vi "pp2_DAQwriteAudioStimulus.vi"(0 "State Info In":T4={"Curr  tr"=0, "Curr (ms)"=0, "Cum (ms)"=0, "Run loop diff"=0, "Tone countdown (ms)"=0, "Countdown (ms)"=0, "Curr State"=enum."0 NULL", "Prev State"=enum."1 Habituation", "Null"=FALSE, "Sw"=FALSE, "Tone\nGate"=FALSE, "Stim"=FALSE, "Current DAQ DO Int"=0, "Current Loaded Trial"={"Trial Type Number"=1, "Trial Type"=enum."GO", "Trial Weight"=100, "Shock (mA)"=0.3, "Duration (ms)"=0.25, "Sound Type"=enum."04 FM Sweep", "Stim P1"=4000.0, "Stim P2"=0.0, "Stim P3"=0.0, "Stim P4"=2000.0}, "Next Trial (for display purposes)"={"Trial Type Number"=1, "Trial Type"=enum."GO", "Trial Weight"=100, "Shock (mA)"=0.3, "Duration (ms)"=0.25, "Sound Type"=enum."04 FM Sweep", "Stim P1"=4000.0, "Stim P2"=0.0, "Stim P3"=0.0, "Stim P4"=2000.0}, "Total trials memo"=0, "State start cum memo (ms)"=0, "Last dur jump time memo (ms)"=0, "Last dur shock time memo (ms)"=0, "Tone repeat memo (ms)"=0, "Webcam on"=FALSE, "Webcam recording"=FALSE} {"Current DAQ DO Int" format="%b"; "Next Trial (for display purposes)"."Shock (mA)" min=-1.0 max=5.0; "Next Trial (for display purposes)"."Trial Weight" step=1; "Next Trial (for display purposes)"."Duration (ms)" min=0.0 max=1.0; "Next Trial (for display purposes)"."Trial Type Number" min=1 step=1; "Current Loaded Trial"."Shock (mA)" min=-1.0 max=5.0; "Current Loaded Trial"."Trial Weight" step=1; "Current Loaded Trial"."Duration (ms)" min=0.0 max=1.0; "Current Loaded Trial"."Trial Type Number" min=1 step=1}, 5 "Daq config In":T1={"Sound AO"="Dev2/ao0", "Shock intesity AO"="Dev1/ao1", "Code_LED DO"="Dev1/port1:2", "Switch DI"="Dev1/port0/line0:1", "Webcam"="cam0", "Sound AO task"="", "Sound card task"=0, "Shock intensity AO task"="", "Code_LED DO task"="", "Switch DI task"="", "AO <=> Sound card"=FALSE, "Sound card"=0, "sample rate"=8000.0, "Variable shock"=FALSE, "Webcam on"=FALSE, "Tone gate PFI"="/Dev1/PFI1", "Waveform memo"={"t0"=timestamp(0 s since 1904-01-01), "dt"=1.0, "Y"=[]}} {"sample rate" min=8000.0; "Sound card task" format="%.0x"}, 11 "error in (no error)":errorcluster) -> (6 "Daq config Out":T1={"Sound AO"="Dev2/ao0", "Shock intesity AO"="Dev1/ao1", "Code_LED DO"="Dev1/port1:2", "Switch DI"="Dev1/port0/line0:1", "Webcam"="cam0", "Sound AO task"="", "Sound card task"=0, "Shock intensity AO task"="", "Code_LED DO task"="", "Switch DI task"="", "AO <=> Sound card"=FALSE, "Sound card"=0, "sample rate"=8000.0, "Variable shock"=FALSE, "Webcam on"=FALSE, "Tone gate PFI"="/Dev1/PFI1", "Waveform memo"={"t0"=timestamp(0 s since 1904-01-01), "dt"=1.0, "Y"=[]}} {"sample rate" min=8000.0; "Sound card task" format="%.0x"}, 15 "error out":errorcluster)   [LabVIEW 2013]
uses:
  pp2_CTL_StateInfo.ctl
  pp2_CTL_State.ctl
  pp2_Trial.ctl
  pp2_CTL_TrialType.ctl
  labolabo2/waveforms/WFTypes.ctl
  pp2_CTL_DaqConfig.ctl
  <vilib>/userdefined/High Color/IMAQdx.ctl
  <vilib>/sound2/lvsound2.llb/Sound Output Task ID.ctl
  labolabo2/waveforms/WFParameters.ctl
  labolabo2/waveforms/WFRepetitions.ctl
  <vilib>/Analysis/NI_AALBase.lvlib
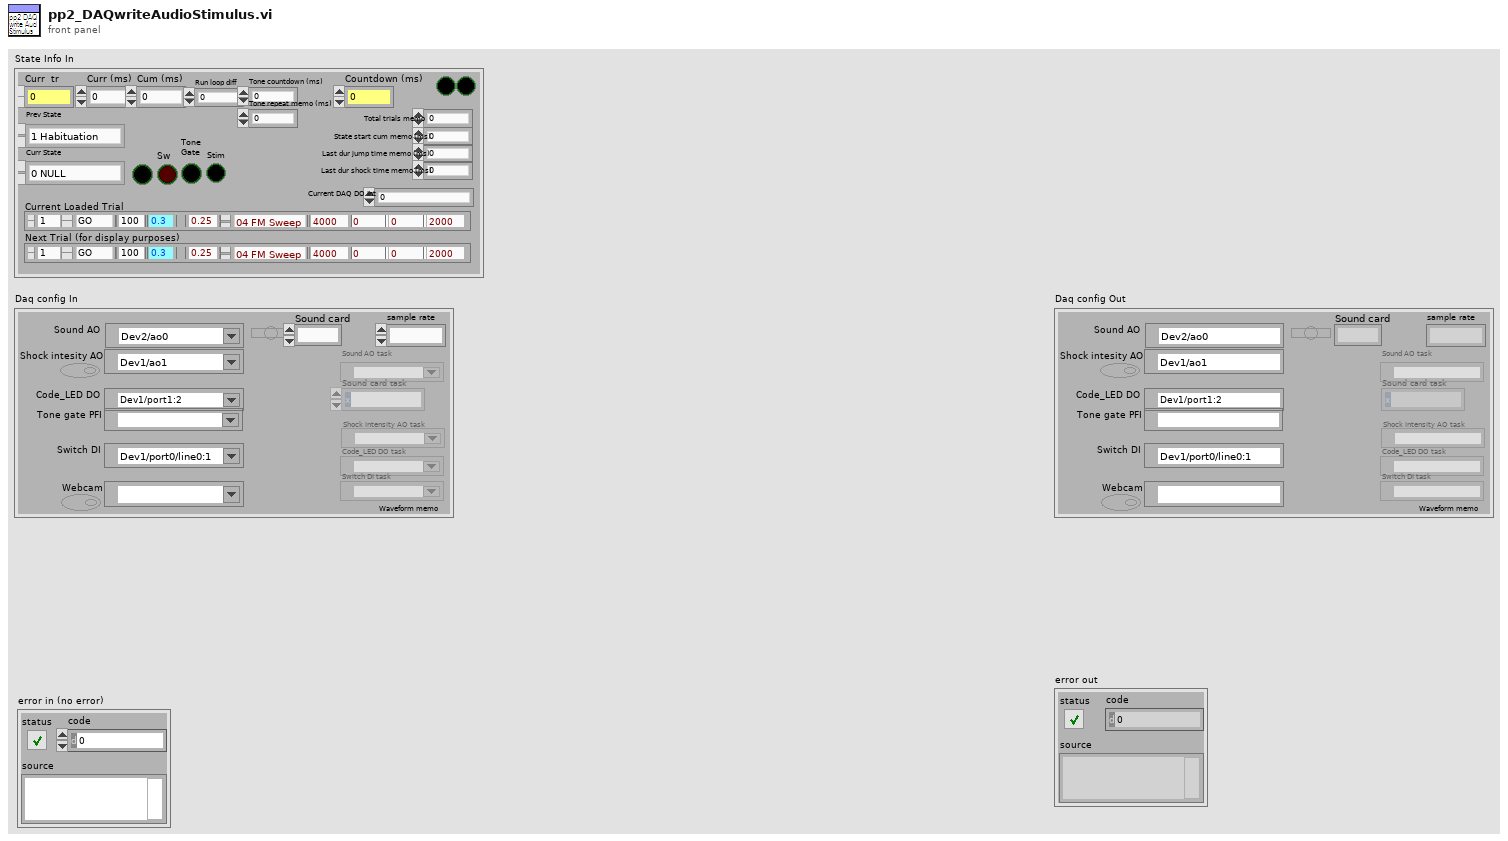
[diagram p1: front panel]
types:
  T1 = typedef "pp2_CTL_DaqConfig.ctl" = cluster{"Sound AO":tag, "Shock intesity AO":tag, "Code_LED DO":tag, "Switch DI":tag, "Webcam":T2, "Sound AO task":refnum<k21>, "Sound card task":T3, "Shock intensity AO task":refnum<k21>, "Code_LED DO task":refnum<k21>, "Switch DI task":refnum<k21>, "AO <=> Sound card":bool, "Sound card":u32, "sample rate":dbl, "Variable shock":bool, "Webcam on":bool, "Tone gate PFI":tag, "Waveform memo":waveform(dbl)}
  T2 = typedef "IMAQdx.ctl" = refnum<k21>
  T3 = typedef "Sound Output Task ID.ctl" = u32
  T4 = typedef "pp2_CTL_StateInfo.ctl" = cluster{"Curr  tr":u16, "Curr (ms)":u32, "Cum (ms)":i64, "Run loop diff":i64, "Tone countdown (ms)":i64, "Countdown (ms)":i64, "Curr State":T5, "Prev State":T5, "Null":bool, "Sw":bool, "Tone\nGate":bool, "Stim":bool, "Current DAQ DO Int":u16, "Current Loaded Trial":T6, "Next Trial (for display purposes)":T6, "Total trials memo":i64, "State start cum memo (ms)":i64, "Last dur jump time memo (ms)":i64, "Last dur shock time memo (ms)":i64, "Tone repeat memo (ms)":i64, "Webcam on":bool, "Webcam recording":bool}
  T5 = typedef "pp2_CTL_State.ctl" = enum8{"0 NULL", "1 Habituation", "2 (Load Trial)", "3 Stay Period", "4 Load Audio/Click Delay", "5 GO Trial", "6 GO Jumped", "7 GO Timeout", "8 NOGO Trial", "9 NOGO Jumped", "10 NOGO Timeout", "11 TEST Trial", "12 TEST Jumped", "13 TEST Timeout", "14 Intertrial Interval", "15 Done"}
  T6 = typedef "pp2_Trial.ctl" = cluster{"Trial Type Number":u8, "Trial Type":T7, "Trial Weight":u32, "Shock (mA)":dbl, "Duration (ms)":dbl, "Sound Type":T8, "Stim P1":dbl, "Stim P2":dbl, "Stim P3":dbl, "Stim P4":dbl}
  T7 = typedef "pp2_CTL_TrialType.ctl" = enum16{"OFF", "GO", "NOGO", "TEST"}
  T8 = typedef "WFTypes.ctl" = enum16{"00 NULL", "01 DC", "02 Noise", "03 Pure Tone", "04 FM Sweep"}
  T9 = typedef "WFRepetitions.ctl" = cluster{"Del (s)":dbl, "Int (s)":dbl, "N":i32}
  T10 = typedef "WFParameters.ctl" = cluster{"Fs (Hz)":dbl, "Amp (V)":dbl, "Ramp (s)":dbl, "Dur (s)":dbl}
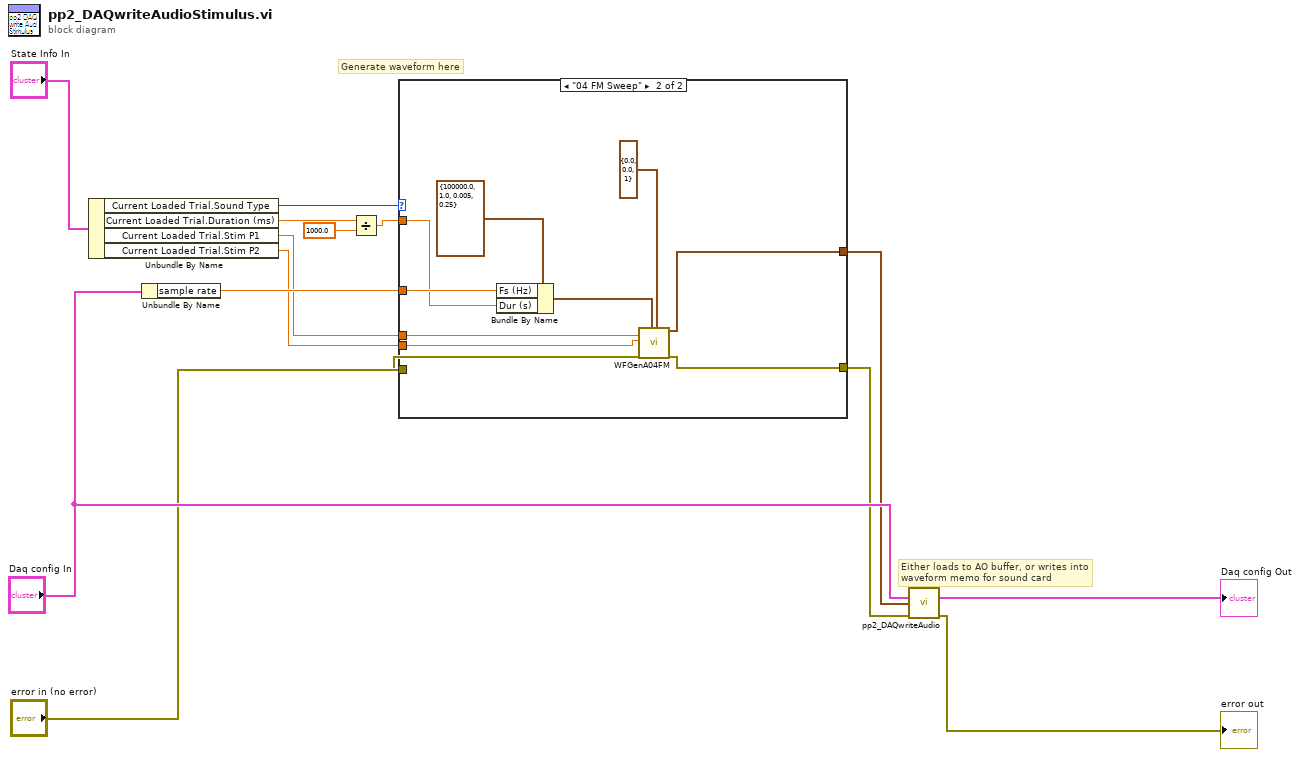
[diagram p0: block diagram]
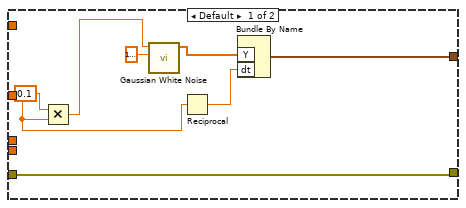
[diagram p2: hidden frame]
diagram:
  # "Either loads to AO buffer, or writes into\nwaveform memo for sound card"
  # "Generate waveform here"
  n1 = Unbundle By Name("State Info In") -> ("Current Loaded Trial.Sound Type"=w13:T8, "Current Loaded Trial.Duration (ms)"=w3:dbl, "Current Loaded Trial.Stim P1"=w5:dbl, "Current Loaded Trial.Stim P2"=w4:dbl)
  n2 = Unbundle By Name("Daq config In") -> ("sample rate"=w12:dbl)
  n3 = Divide(x=w3, y=1000.0) -> (x/y=w2:dbl)
  n4 = case shown="\"04 FM Sweep\"" w13 {
    tunnel: w12 -> [w17 w31]
    tunnel: [w16 w24] -> w7
    tunnel: "error in (no error)" -> [w15 w25]
    tunnel: [w15 w23] -> w9
    tunnel: w2 -> [_ w28]
    tunnel: w5 -> [_ w27]
    tunnel: w4 -> [_ w26]
    frame Default {
      n5 = Multiply(x=0.1, y=w17) -> (x*y=w20:dbl)
      n6 = call <vilib>:"Gaussian White Noise.vi"("standard deviation"=1.0000000000000002, "samples"=w20) -> ("Gaussian noise pattern"=w19:dbl[])  [unwired: 8 in, 1 out]
      n7 = Reciprocal(x=w17) -> (1/x=w18:dbl)
      n8 = Bundle By Name("Y"=w19, "dt"=w18) -> (w16:waveform(dbl))  [unwired: 1 in]
    }
    frame "04 FM Sweep" {
      n9 = Bundle By Name(cluster=T10 {"Fs (Hz)"=100000.0, "Amp (V)"=1.0, "Ramp (s)"=0.005, "Dur (s)"=0.25} ("WFParameters"), "Fs (Hz)"=w31, "Dur (s)"=w28) -> (w29:T10)
      n10 = call "WFGenA04FM.vi"("Param 0: Start Hz"=w27, "Param 1: End Hz"=w26, "error in (no error)"=w25, "WFParameters"=w29, "WFRepetitions"=T9 {"Del (s)"=0.0, "Int (s)"=0.0, "N"=1}) -> ("Waveform Out"=w24:waveform(dbl), "error out"=w23:errorcluster)  [unwired: 13 in]
    }
  }
  n11 = call "pp2_DAQwriteAudio.vi"("Daq config In"="Daq config In", "Waveform"=w7, "error in (no error)"=w9) -> ("Daq config Out"=→"Daq config Out":T1, "error out"=→"error out":errorcluster)  [unwired: 11 in]
